vi "Tear Down.vi"(8 "error in (no error)":errorcluster, 11 "Terminal Message in":refnum<class "Terminal Message.lvclass">) -> (0 "error out":errorcluster, 3 "Terminal Message out":refnum<class "Terminal Message.lvclass">)   [LabVIEW 2016, in "CLD Exam - ATM.lvlib" / "Terminal Message.lvclass"]
uses:
  Terminal Message.lvclass
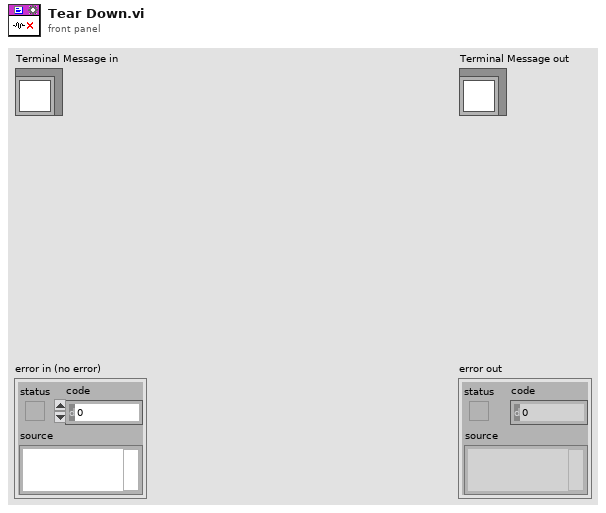
[diagram p1: front panel]
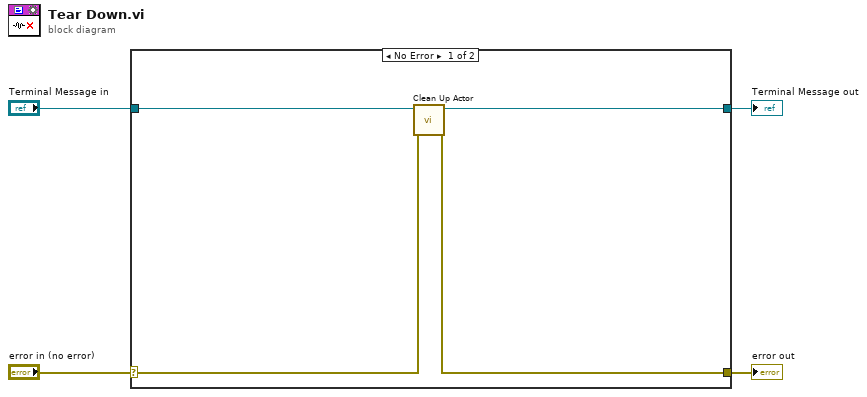
[diagram p0: block diagram]
diagram:
  n1 = case shown="No Error" "error in (no error)" {
    selector: "error in (no error)" -> [w6 w10]
    tunnel: [w5 w10] -> w3
    tunnel: [w7 w9] -> w1
    tunnel: "Terminal Message in" -> [w8 w9]
    frame No Error {
      n2 = call-dynamic "Clean Up Actor.vi"("error in (no error)"=w6, "Terminal Message in"=w8) -> ("error out"=w5:errorcluster, "Terminal Message out"=w7:refnum<class "Terminal Message.lvclass">)  [unwired: 8 in]
    }
    frame Error {
    }
  }
  "error out" <- w3
  "Terminal Message out" <- w1
